vi "MobileTest_DUTConfigure.vi"() -> ()   [LabVIEW 2019]
uses:
  Public/Documents/National Instruments/TestStand 2019 (64-bit)/Examples/Demos/Mobile Device Test/LabVIEW/Source/Support/Simulation Data.ctl
  Public/Documents/National Instruments/TestStand 2019 (64-bit)/Examples/Demos/Mobile Device Test/LabVIEW/Source/Support/Wifi Test Modes.ctl
panel:
  out "QAM Data Received":cluster{dbl[], dbl[]}[](graph)
  in  "Mode List":T1[](array[typedef])
  out "QAM Data Transmitted":cluster{dbl[], dbl[]}[](graph)
  in  "Simulation Data":T2={"PowerOn"=TRUE, "Battery"=TRUE, "Antenna"=TRUE, "Microphone"=TRUE, "Speakers"=TRUE, "Buttons"=TRUE, "LCD"=enum."Passing Image"}
  out "Error Out":errorcluster
  in  "Transmitted Data String":string="1. Generate System Parameters.  This VI generates a symbol map and computes bits per symbol for the given QAM selection.\n2. Bit Coding.  This VI converts an array of U8 characters into a binary array, adding Log2(M) guard bits to the front of the bistream.\n3. Generate Filter Coefficients.  Generates pulse shaping and matching filter coefficients\n4. Modulate QAM.  Converts the bitstream into an array of IQ values.\n5. Add AWGN.  This VI adds impairments such as increasing the noise floor of the signal\n    (note, steps 6 and 7 are used only for visualization/analysis purposes)\n6. Upconversion.  Converts an array of IQ values into a waveform based on the carrier frequency\n7. Spectral Measurements.  Performs an FFT of the upconverted waveform to illustrate the carrier band.\n8. Demodulate QAM.  Conerts an array of IQ values into a bitstream\n    (note, step 9 is used only for visualization/analysis purposes)\n9. Format Constillation Plot.  Generate a constilation plot for the demodulated IQ data.\n10. Convert the bistream into an array of U8's, so that that the resulting information can be viewed in character format.\n\nqwertyuiop[asdfghjkl;xcvbnm,./\n"
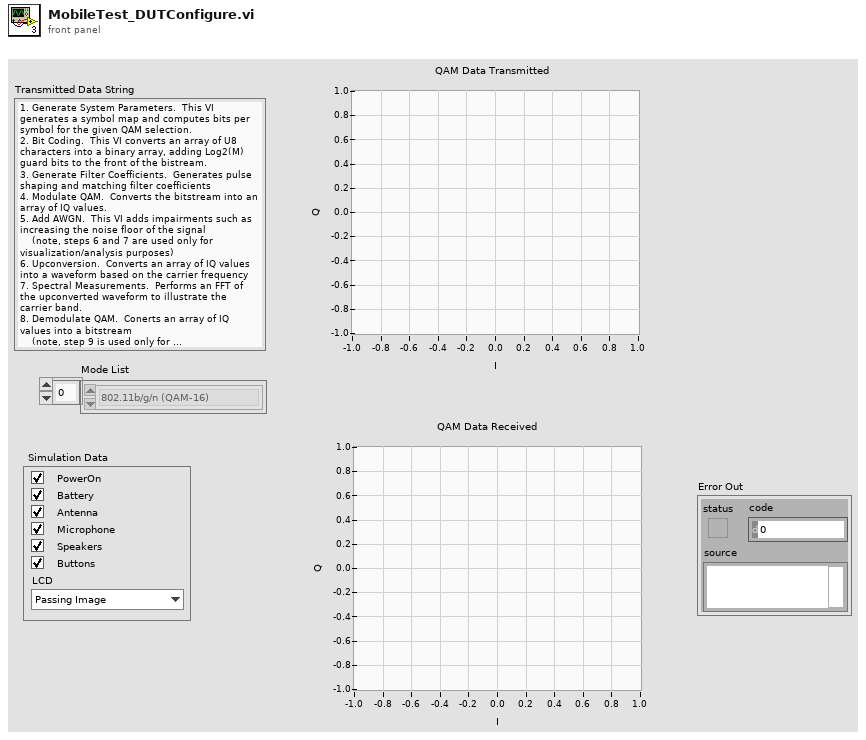
[diagram p1: front panel]
types:
  T1 = typedef "Wifi Test Modes.ctl" = enum16{"802.11b/g/n (QAM-16)", "LTE (QAM-64)", "802.11ac (QAM-256)"}
  T2 = typedef "Simulation Data.ctl" = cluster{"PowerOn":bool, "Battery":bool, "Antenna":bool, "Microphone":bool, "Speakers":bool, "Buttons":bool, "LCD":enum16{"Passing Image", "Dead Pixels", "Incorrect Brightness"}}
  T3 = cluster{"QAM Data":cluster{dbl[], dbl[]}, "QAM Data Out":cluster{dbl[], dbl[]}, "symbol map 16 QAM":cdb[], "Mode":T1}
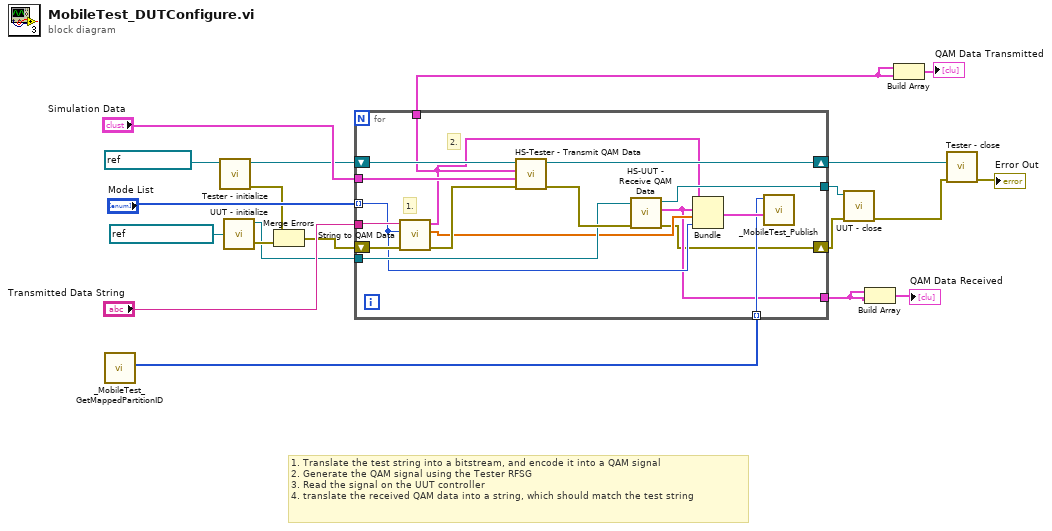
[diagram p0: block diagram]
diagram:
  # "1. Translate the test string into a bitstream, and encode it into a QAM signal\n2. Generate the QAM signal using the Tester RFSG\n3. Read the signal on the UUT controller\n4. translate the received QAM data into a string, which should match the test string"
  n1 = call "_MobileTest_GetMappedPartitionID.vi"() -> ("ID"=w11:u32[])  [unwired: 11 in]
  n2 = call "Tester - initialize.vi"("VISA resource name"=refnum<visa-resource-name> "TesterRFSG") -> ("error out"=w8:errorcluster, "VISA resource name out"=w18:refnum<visa-resource-name>)  [unwired: 9 in]
  n3 = call "UUT - initialize.vi"("VISA resource name"=refnum<visa-resource-name> "UUTController") -> ("error out"=w9:errorcluster, "VISA resource name out"=w6:refnum<visa-resource-name>)  [unwired: 9 in]
  n4 = Merge Errors(w8, w9) -> (w7:errorcluster)
  n5 = for {
    tunnel: "Simulation Data" -> [w36]
    tunnel: "Mode List" -> [w26] mode=indexing
    tunnel: "Transmitted Data String" -> [w32]
    tunnel: [w21] -> w14
    shift-right: [w33] -> w17
    shift-left: w18 -> [w34]
    shift-right: [w22] -> w4
    shift-left: w7 -> [w31]
    tunnel: w11 -> [w25] mode=indexing
    tunnel: w6 -> [w29]
    tunnel: [w24] -> w5
    tunnel: [w23] -> w2
    # "2."
    # "1."
    n6 = call "String to QAM Data.vi"("error in (no error)"=w31, "Mode"=w26, "Transmitted Data String"=w32) -> ("error out"=w35:errorcluster, "symbol map 16 QAM"=w27:cdb[], "QAM Data"=w21:cluster{dbl[], dbl[]})  [unwired: 6 in]
    n7 = call "HS-Tester - Transmit QAM Data.vi"("error in (no error)"=w35, "Simulation Data"=w36, "QAM Data In"=w21, "VISA resource name"=w34) -> ("error out"=w30:errorcluster, "VISA resource name out"=w33:refnum<visa-resource-name>)  [unwired: 6 in]
    n8 = call "HS-UUT - Receive QAM Data.vi"("error in (no error)"=w30, "VISA resource name"=w29) -> ("error out"=w22:errorcluster, "QAM Data Out"=w23:cluster{dbl[], dbl[]}, "VISA resource name out"=w24:refnum<visa-resource-name>)  [unwired: 7 in]
    n9 = Bundle("QAM Data"=w21, "QAM Data Out"=w23, "symbol map 16 QAM"=w27, "Mode"=w26) -> (w28:T3)  [unwired: 1 in]
    n10 = call "_MobileTest_Publish.vi"("Data"=w28, "id"=w25) -> ()  [unwired: 9 in]
  }
  n11 = call "UUT - close.vi"("error in (no error)"=w4, "VISA resource name"=w5) -> ("error out"=w3:errorcluster)  [unwired: 9 in]
  n12 = Build Array(w2, w2) -> (→"QAM Data Received":cluster{dbl[], dbl[]}[])
  n13 = Build Array(w14, w14) -> (→"QAM Data Transmitted":cluster{dbl[], dbl[]}[])
  n14 = call "Tester - close.vi"("error in (no error)"=w3, "VISA resource name"=w17) -> ("error out"=→"Error Out":errorcluster)  [unwired: 9 in]
